vi "ADQ214 Get Acquired All.vi"(8 "error in":errorcluster, 11 "adq_cu_ptr":u32) -> (0 "error out":errorcluster, 2 "return":u32, 3 "adq_cu_ptr":u32)   [LabVIEW 2013]
uses:
  GetData_DLL.dll
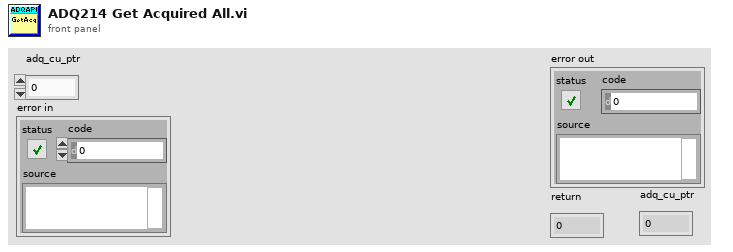
[diagram p1: front panel]
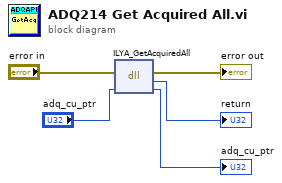
[diagram p0: block diagram]
diagram:
  n1 = dll-call lib="C:/Users/astafiev/Desktop/Ilya/LabView_Imperium/GetData_DLL.dll" fn="ILYA_GetAcquiredAll"(error in="error in", "adq_cu_ptr"="adq_cu_ptr") -> (error out=→"error out":errorcluster, "return type"=→"return":u32, "adq_cu_ptr"=→"adq_cu_ptr":u32)  [unwired: 2 in, 1 out]
